vi "표지판.vi"() -> ()   [LabVIEW 2018]
panel:
  out "좌측차선 U 3":dbl
  out "좌측차선 U 2":dbl
  out "좌측차선 U":dbl
  out "반환값":i32
  in  "정지":bool
  out "에러 출력":errorcluster caption="에러 1"
  in  "function_1":string
  in  "1st module":path
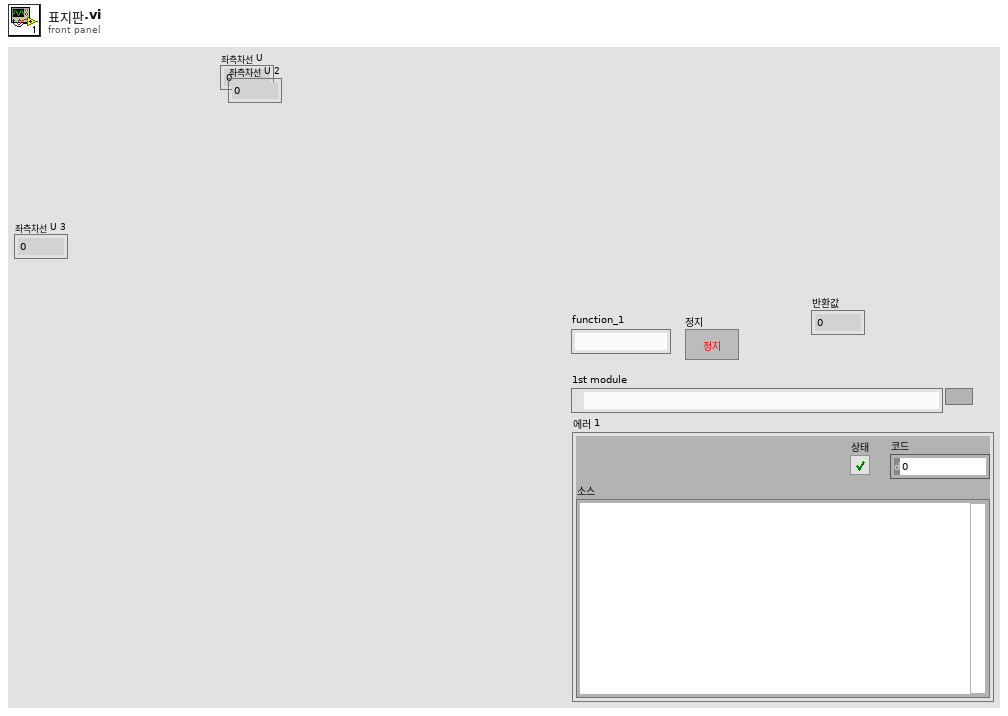
[diagram p1: front panel]
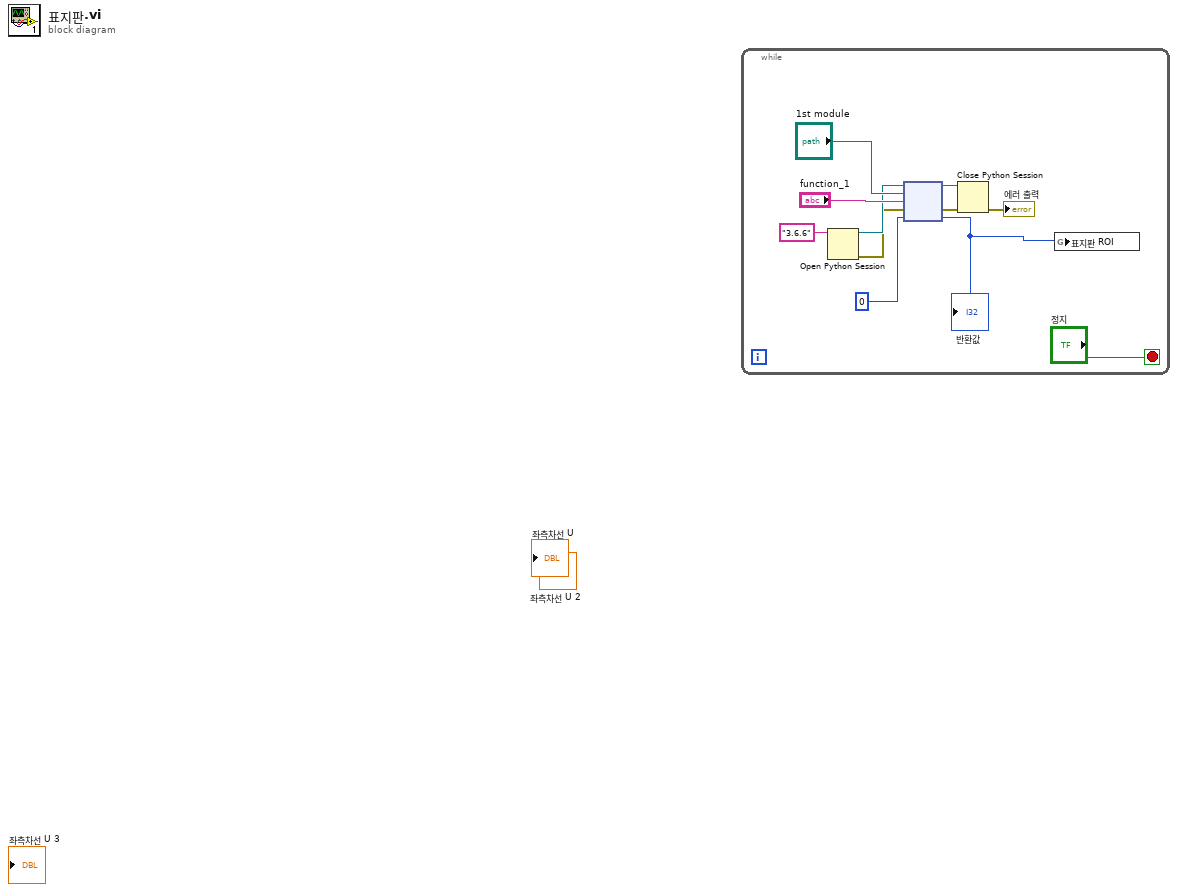
[diagram p0: block diagram]
diagram:
  n1 = while {
    stop <- "정지" stop-if-true
    n2 = Open Python Session(python version="3.6.6" ("Python 버전")) -> (session out=w6:refnum<k35>, error out=w5:errorcluster)  [unwired: 2 in]
    n3 = node(w6, "1st module", "function_1", w5, 0) -> (w10:refnum<k35>, w7:errorcluster, w2:i32)  [unwired: 2 out]
    "반환값" <- w2
    n4 = Close Python Session(session in=w10, error in=w7) -> (11:→"에러 출력":errorcluster)
    n5 = global write "빨간불.vi" "표지판 ROI"(w2) -> ()
  }
